vi "AAA MotorTestBench.vi"() -> ()   [LabVIEW 2020]
uses:
  <instrlib>/Gantner Instruments/Ethernet/Gantner-Instruments HighSpeedPort.llb/e.gate Protocol Type.ctl
  <vilib>/Instr/_visa.llb/VISA Configure Serial Port (Instr).vi
  <vilib>/Utility/file.llb/Write Delimited Spreadsheet (string).vi
panel:
  out "Humidity (%)":string
  out "Pressure (Pa)":string
  out "Temperature (°C)":string
  out "Elapsed Time":string
  out "?":dbl[](array[slide]) scale=0.0..1000.0
  out "Temperature 2":dbl[](array[slide]) caption="Thermocouple 1" scale=20.0..50.0
  out "error out 2":errorcluster
  in  "?":bool
  out "Random Number":dbl(knob) scale=0.0..180.0
  out "error out":errorcluster
  in  "START":bool
  out "PWM Feedback":string
  in  "PWM Value":string
  # "Hacker A150-12  -  Motor control"
  # "Temperatures"
  # "Torque"
  # "Vibration"
  # "Power Supply"
  # "Atmospheric\nConditions"
  # "Voltage"
  # "Thrust"
  # "Current"
  # "Battery Data"
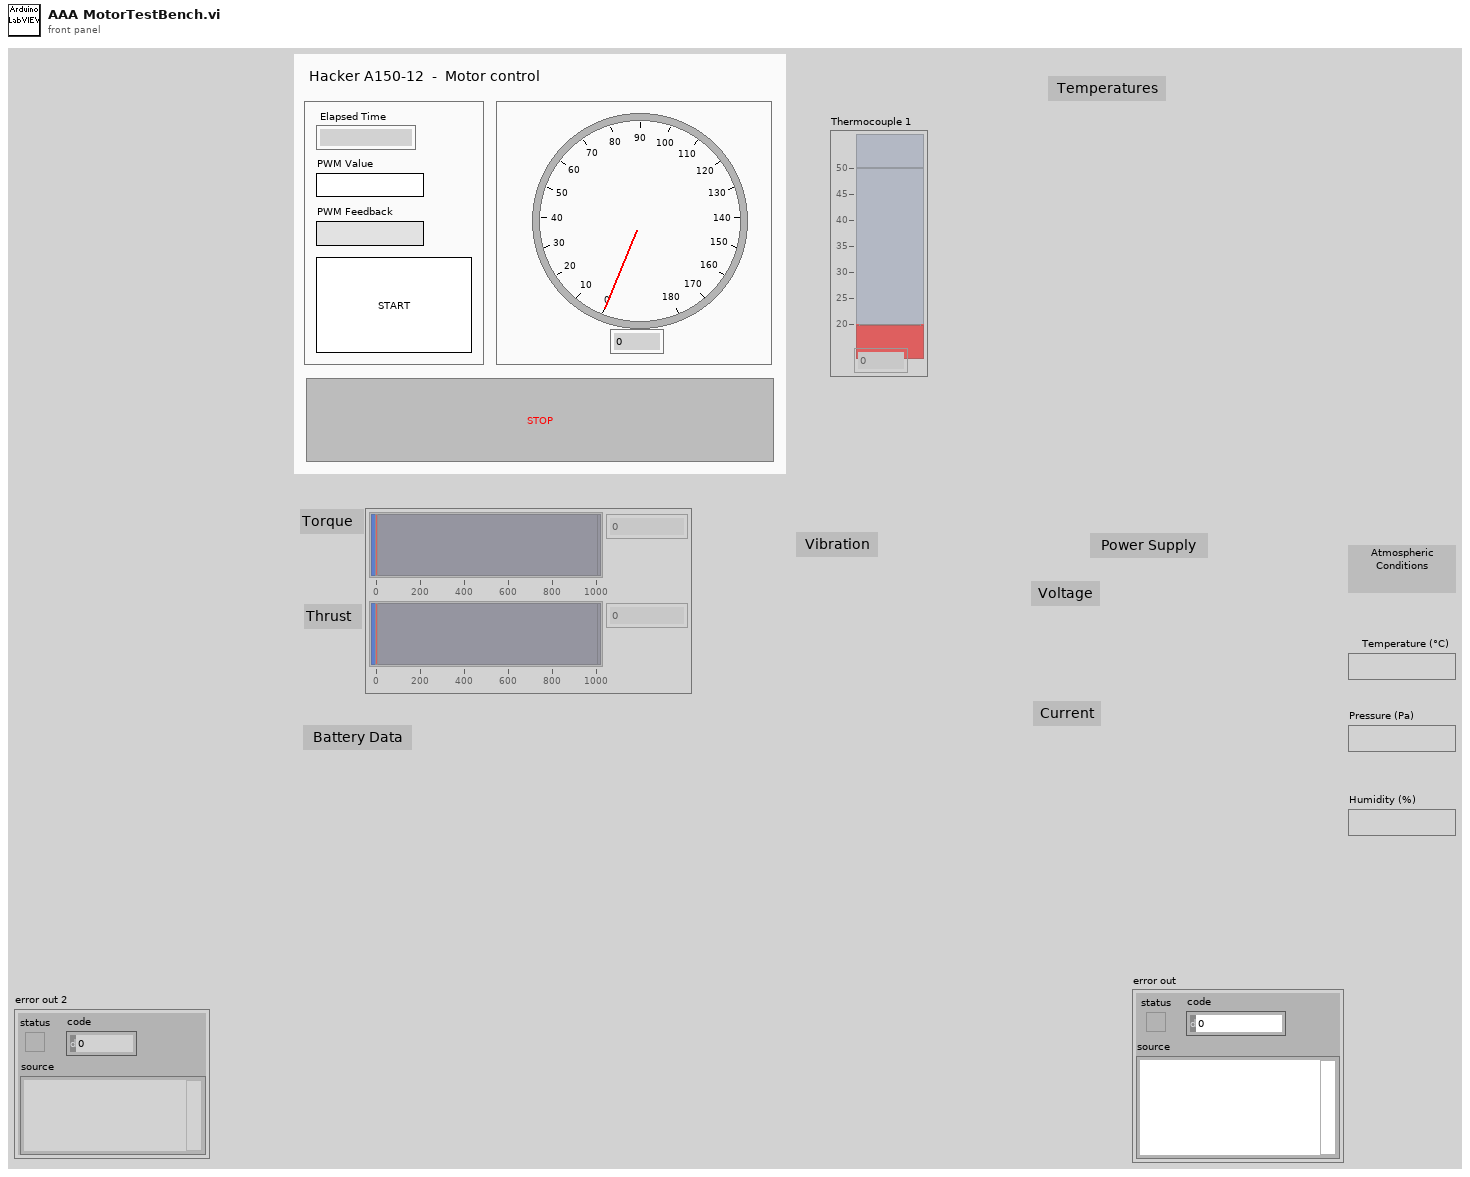
[diagram p1: front panel]
types:
  T1 = typedef "e.gate Protocol Type.ctl" = enum16{"ASCII", "HighspeedPort Online", "HighspeedPort Buffer (giutility.DLL) ", "PostProcessBuffer (giutility.DLL)", "HighspeedPort Online (giutility.DLL)", "Decode UDBF File (giutility.DLL)"}
  T2 = typedef "e.gate Configuration.ctl" = cluster{"connection ID":refnum<k5>, "IPAddress":string, "BufferIndex":i32, "StateMessage":string, "StateCode":i8, "HeaderSize":i32, "BufferSize":i32, "IsBigEndian":i32, "Version":i32, "ChannelCount":i32, "FrameLength":i32, "StartTime":dbl, "dActTimeToSecondFactor":dbl, "StartTimeToDayFactor":dbl, "BufferFillRate":dbl, "SampleRate":dbl, "ChannelData":T3[], "DecodeTimeFormat":string, "SummaryPath":string, "WithCheckSum":i32, "dActTimeDataType":T4, "MaxWriteCount":i32, "MaxReadCount":i32, "TempOffsetRead":i32, "TempLengthRead":i32, "Protocol":T1, "IsSupported":i32, "InputAccessList":i32[], "OutputAccessList":i32[], "DataSource":enum16{"CircleBuffer", "test.con Logger", "test.con Archive"}, "Modules":T5[], "DLL-Handle":T6}
  T3 = typedef "e.gate Channel Data.ctl" = cluster{"VariableName":string, "DataDirection":string, "DataType":string, "DataTypeIndex":T4, "Precision":i16, "FieldLengtht":i16, "ByteCount":i32, "Format":string, "Unit":string, "InputAccessOffset":i32, "OutputAccessOffset":i16, "InputAccessIndex":i16, "OutputAccessIndex":i16, "VarType":string}
  T4 = typedef "e.gate Data Type.ctl" = enum16{"NO", "BOOL", "SINT8", "USINT8", "SINT16", "USINT16", "SINT32", "USINT32", "FLOAT", "SET8", "SET16", "SET32", "DOUBLE", "SINT64", "USINT64", "SET64"}
  T5 = typedef "e.gate Module  Data.ctl" = cluster{"Type":string, "Location":string, "VariablesCount":i16, "UartIndex":i16, "Address":i16, "SystemOffset":i16}
  T6 = typedef "e.gateHSP_DLLhandle.ctl" = cluster{"clientInstance":i32, "connectionInstance":i32, "Is32Bit":bool, "DLL Path":path}
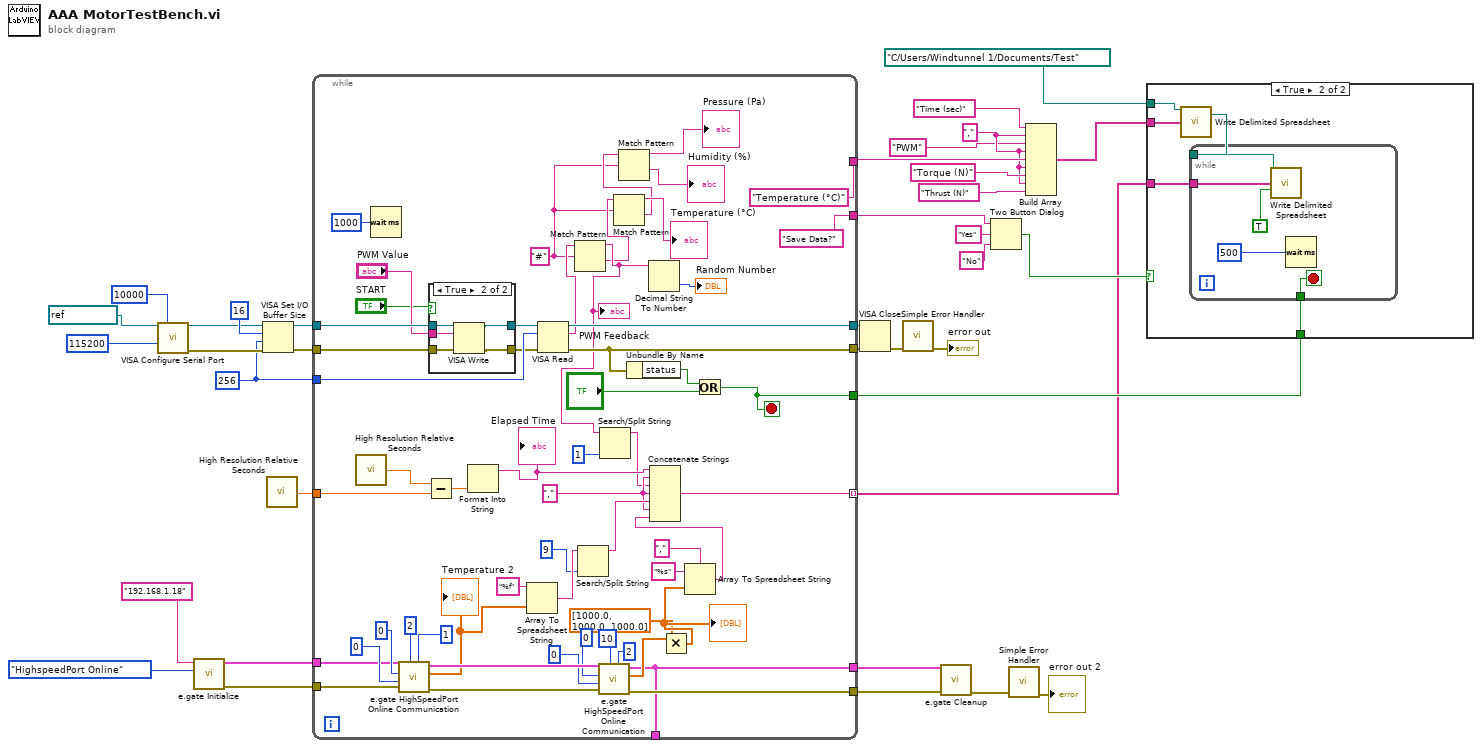
[diagram p0: block diagram]
diagram:
  w2 = "," ("element")
  w24 = u32 256 ("buffer size")
  n1 = call-poly "VISA Configure Serial Port"("VISA resource name"=refnum<visa-resource-name> "COM5", "timeout (10sec)"=u32 10000, "baud rate (9600)"=u32 115200) -> ("VISA resource name out"=w33:refnum<visa-resource-name>, "error out"=w32:errorcluster)  [unwired: 11 in]
  n2 = call <instrlib>:"e.gate Initialize.vi"("Protocol"=e.gate_Protocol_Type."HighspeedPort Online", "IP Address"="192.168.1.18") -> ("error out"=w18:errorcluster, "e.gate Configuration"=w19:T2)  [unwired: 8 in]
  n3 = VISA Set I/O Buffer Size(VISA resource name=w33, mask (16)=u16 16 ("I/O Receive\nBuffer mask"), size (4096)=w24, error in (no error)=w32) -> (VISA resource name out=w31:refnum<visa-resource-name>, error out=w30:errorcluster)
  n4 = call <vilib>:"High Resolution Relative Seconds.vi"() -> ("relative seconds"=w7:dbl)
  n5 = while {
    tunnel: w31 -> [w91]
    tunnel: w30 -> [w90]
    tunnel: [w92] -> w36
    tunnel: [w83] -> w35
    tunnel: w24 -> [w93]
    tunnel: w19 -> [w70]
    tunnel: w18 -> [w69]
    tunnel: [w37] -> w17
    tunnel: [w68] -> w16
    tunnel: ["Save Data?" ("message")] -> w11
    tunnel: [w66] -> w10
    tunnel: ["Temperature (°C)" ("element")] -> w9
    tunnel: w7 -> [w62]
    tunnel: [w58] -> w8 mode=indexing
    tunnel: [w37] -> _
    stop <- w66 stop-if-true
    w43 = "#" ("regular expression")
    w51 = "," ("string")
    n6 = call <vilib>:"High Resolution Relative Seconds.vi"() -> ("relative seconds"=w63:dbl)
    n7 = Wait (ms)(milliseconds to wait=u32 1000) -> ()  [unwired: 1 out]
    n8 = call <instrlib>:"e.gate HighSpeedPort Online Communication.vi"("ReadCount"=1, "ReadIndex"=2, "error in (no error)"=w69, "WriteCount"=0, "WriteIndex"=0, "e.gate Configuration In"=w70) -> ("error out"=w75:errorcluster, "Value"=w64:dbl[], "e.gate Configuration Out"=w76:T2)  [unwired: 3 in]
    "Temperature 2" <- w64
    n9 = Subtract(x=w63, y=w62) -> (x-y=w61:dbl)
    n10 = case shown="True" "START" {
      tunnel: w91 -> [w95 w100]
      tunnel: w90 -> [w94 w99]
      tunnel: [w95 w98] -> w89
      tunnel: [w94 w97] -> w88
      tunnel: "PWM Value" -> [_ w96]
      frame False {
      }
      frame True {
        n11 = VISA Write(VISA resource name=w100, write buffer=w96, error in (no error)=w99) -> (VISA resource name out=w98:refnum<visa-resource-name>, error out=w97:errorcluster)  [unwired: 1 out]
      }
    }
    n12 = Format Into String(w61) -> (resulting string=w52:string)  [unwired: 3 in, 1 out]
    "Elapsed Time" <- w52
    n13 = Array To Spreadsheet String(array=w64, 3:"%f" ("format string")) -> (spreadsheet string=w55:string)  [unwired: 1 in]
    n14 = VISA Read(VISA resource name=w89, byte count=w93, error in (no error)=w88) -> (VISA resource name out=w92:refnum<visa-resource-name>, read buffer=w48:string, error out=w83:errorcluster)  [unwired: 1 out]
    n15 = Match Pattern(string=w48, regular expression=w43) -> (before substring=w47:string, after substring=w46:string)  [unwired: 1 in, 2 out]
    "PWM Feedback" <- w47
    n16 = Search/Split String(string=w55, offset (0)=9) -> (substring before match=w54:string)  [unwired: 1 in, 2 out]
    n17 = call <instrlib>:"e.gate HighSpeedPort Online Communication.vi"("ReadCount"=2, "ReadIndex"=10, "error in (no error)"=w75, "WriteCount"=0, "WriteIndex"=0, "e.gate Configuration In"=w76) -> ("error out"=w68:errorcluster, "Value"=w40:dbl[], "e.gate Configuration Out"=w37:T2)  [unwired: 3 in]
    n18 = Search/Split String(string=w47, offset (0)=1) -> (substring before match=w50:string)  [unwired: 1 in, 2 out]
    n19 = Match Pattern(string=w46, regular expression=w43) -> (before substring=→"Temperature (°C)":string, after substring=w44:string)  [unwired: 1 in, 2 out]
    n20 = Match Pattern(string=w44, regular expression=w43) -> (before substring=→"Pressure (Pa)":string, after substring=→"Humidity (%)":string)  [unwired: 1 in, 2 out]
    n21 = Unbundle By Name(w83) -> ("status"=w82:bool)
    n22 = Decimal String To Number(string=w47) -> (number=→"Random Number":i32)  [unwired: 2 in, 1 out]
    n23 = Multiply(x=w40, y=dbl[] [1000.0, 1000.0, 1000.0]) -> (x*y=w39:dbl[])
    "?" <- w39
    n24 = Array To Spreadsheet String(delimiter (Tab)=",", array=w39, 3:"%s" ("format string")) -> (spreadsheet string=w56:string)
    n25 = Concatenate Strings(w52, w51, w50, w51, w54, w51, w56) -> (w58:string)
    n26 = Or(x=w82, y="?") -> (x .or. y?=w66:bool)
  }
  n27 = VISA Close(VISA resource name=w36, error in (no error)=w35) -> (error out=w29:errorcluster)
  n28 = call <vilib>:"Simple Error Handler.vi"("error in (no error)"=w29) -> ("error out"=→"error out":errorcluster)  [unwired: 4 in, 4 out]
  n29 = call <instrlib>:"e.gate Cleanup.vi"("error in (no error)"=w16, "e.gate Configuration"=w17) -> ("error out"=w23:errorcluster)  [unwired: 9 in]
  n30 = Two Button Dialog(message=w11, 1:"No" ("F button name (\"Cancel\")"), 2:"Yes" ("T button name (\"OK\")")) -> (T button?=w14:bool)
  n31 = call <vilib>:"Simple Error Handler.vi"("error in (no error)"=w23) -> ("error out"=→"error out 2":errorcluster)  [unwired: 4 in, 4 out]
  n32 = Build Array("Time (sec)" ("element"), w2, "PWM" ("element"), w2, w9, w2, "Torque (N)" ("element"), w2, "Thrust (N)" ("element")) -> (w15:string[])
  n33 = case shown="True" w14 {
    tunnel: w15 -> [_ w104]
    tunnel: w10 -> [_ w103]
    tunnel: w8 -> [_ w102]
    tunnel: path "C:/Users/Windtunnel 1/Documents/Test" ("file path (dialog if empty) 2") -> [_ w101]
    frame False {
    }
    frame True {
      n34 = call-poly <vilib>:"Write Delimited Spreadsheet.vi"("file path (dialog if empty)"=w101, "1D data"=w104) -> ("new file path (Not A Path if cancelled)"=w105:path)  [unwired: 12 in, 1 out]
      n35 = while {
        tunnel: w105 -> [w110]
        tunnel: w103 -> [w107]
        tunnel: w102 -> [w106]
        stop <- w107 stop-if-true
        n36 = call-poly <vilib>:"Write Delimited Spreadsheet.vi"("file path (dialog if empty)"=w110, "1D data"=w106, "append to file? (new file:F)"=TRUE) -> ()  [unwired: 11 in, 2 out]
        n37 = Wait (ms)(milliseconds to wait=u32 500) -> ()  [unwired: 1 out]
      }
    }
  }
